vi "Create Menu.vi"(8 "error in (no error)":errorcluster, 9 "Cell Position":T1, 10 "Cell Data":string, 11 "Menu in":refnum<k9>) -> (0 "error out":errorcluster)   [LabVIEW 2021, in "Model_AMC.lvclass"]
uses:
  Model_AMC.lvclass
  <vilib>/Utility/miscctls.llb/LVRowAndColumnTypeDef.ctl
  Model_AMC.lvclass/Model_AMC.ctl
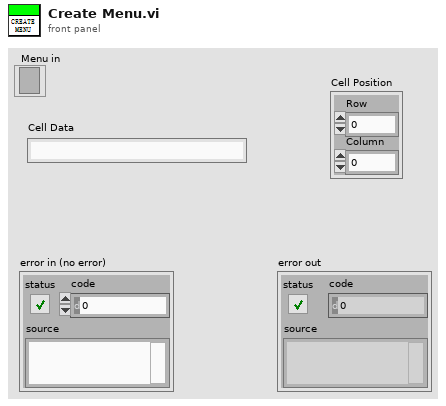
[diagram p1: front panel]
types:
  T1 = typedef "LVRowAndColumnTypeDef.ctl" = cluster{"Row":i32, "Column":i32}
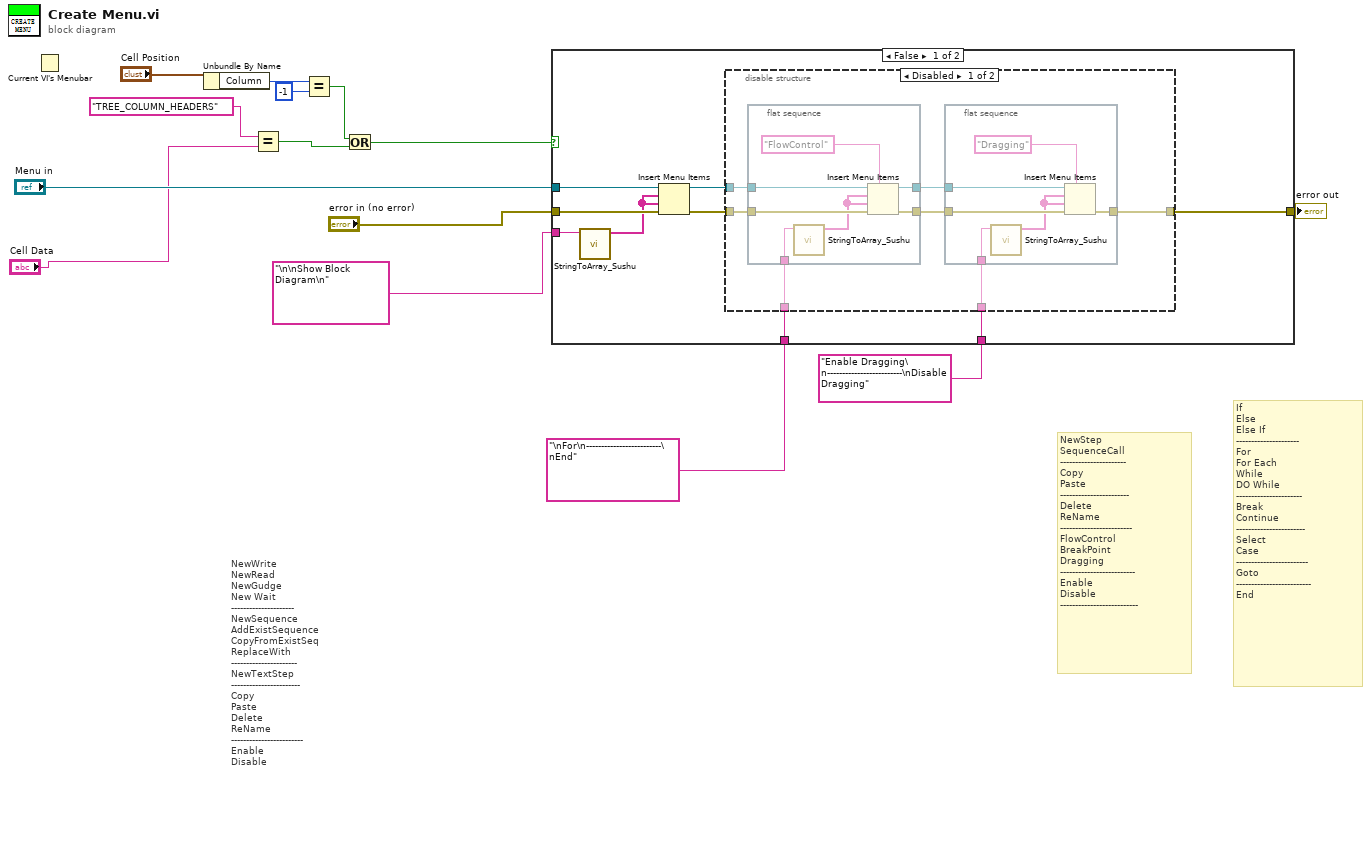
[diagram p0: block diagram]
diagram:
  # "NewStep\nSequenceCall\n----------------------\nCopy\nPaste\n-----------------------\nDelete\nReName\n------------------------\nFlowControl\nBreakPoint\nDragging\n-------------------------\nEnable\nDisable\n--------------------------"
  # "If\nElse\nElse If\n---------------------\nFor\nFor Each\nWhile\nDO While\n----------------------\nBreak\nContinue\n-----------------------\nSelect\nCase\n------------------------\nGoto\n-------------------------\nEnd"
  # "NewWrite\nNewRead\nNewGudge\nNew Wait\n---------------------\nNewSequence\nAddExistSequence\nCopyFromExistSeq\nReplaceWith\n----------------------\nNewTextStep\n-----------------------\nCopy\nPaste\nDelete\nReName\n------------------------\nEnable\nDisable"
  n1 = Current VI's Menubar() -> ()  [unwired: 1 out]
  n2 = Unbundle By Name("Cell Position") -> ("Column"=w7:i32)
  n3 = Equal?(x="TREE_COLUMN_HEADERS", y="Cell Data") -> (x = y?=w11:bool)
  n4 = Equal?(x=w7, y=-1) -> (x = y?=w10:bool)
  n5 = Or(x=w10, y=w11) -> (x .or. y?=w4:bool)
  n6 = case shown="False" w4 {
    tunnel: "Menu in" -> [w23 _]
    tunnel: "error in (no error)" -> [w22 w44]
    tunnel: [w16 w44] -> w12
    tunnel: "\nFor\n-------------------------\nEnd" ("State Queue") -> [w19 _]
    tunnel: "\n\nShow Block Diagram\n" ("State Queue") -> [w18 _]
    tunnel: "Enable Dragging\n-------------------------\nDisable Dragging" ("State Queue") -> [w15 _]
    frame False {
      n7 = call <userlib>:"StringToArray_Sushu.vi"("State Queue"=w18) -> ("Array"=w17:string[])  [unwired: 7 in, 3 out]
      n8 = Insert Menu Items(6:w22, 7:w17, 8:w17, 9:w23) -> (0:w20:errorcluster, 3:w21:refnum<k9>)  [unwired: 2 in, 1 out]
      n9 = disable-structure shown="Disabled" {
        disable-tunnel: w21 -> [w30 _]
        disable-tunnel: w20 -> [w29 _]
        disable-tunnel: w19 -> [w28 _]
        disable-tunnel: [w26 _] -> w16
        disable-tunnel: w15 -> [w24 _]
        frame Disabled {
          n10 = flat-sequence {
            tunnel: w30 -> [w42]
            tunnel: w29 -> [w41]
            tunnel: [w40] -> w27
            tunnel: w28 -> [w39]
            tunnel: [w37] -> w25
            frame #0 {
              n11 = call <userlib>:"StringToArray_Sushu.vi"("State Queue"=w39) -> ("Array"=w38:string[])  [unwired: 7 in, 3 out]
              n12 = Insert Menu Items(5:"FlowControl" ("menu tag"), 6:w41, 7:w38, 8:w38, 9:w42) -> (0:w40:errorcluster, 3:w37:refnum<k9>)  [unwired: 1 in, 1 out]
            }
          }
          n13 = flat-sequence {
            tunnel: w25 -> [w35]
            tunnel: w27 -> [w34]
            tunnel: [w33] -> w26
            tunnel: w24 -> [w32]
            frame #0 {
              n14 = call <userlib>:"StringToArray_Sushu.vi"("State Queue"=w32) -> ("Array"=w31:string[])  [unwired: 7 in, 3 out]
              n15 = Insert Menu Items(5:"Dragging" ("menu tag"), 6:w34, 7:w31, 8:w31, 9:w35) -> (0:w33:errorcluster)  [unwired: 1 in, 2 out]
            }
          }
        }
        frame Enabled {
        }
      }
    }
    frame True {
    }
  }
  "error out" <- w12
